vi "Close.vi"(8 "error in (no error)":errorcluster, 11 "DI (N Samples) Ref In":T1) -> (0 "error out":errorcluster)   [LabVIEW 2021, in "DI Block.lvlib"]
doc: "Closes the reference to one or more digital input channels, sets the logic levels of all digital input channels to low, and disables all digital input channels."
uses:
  <vilib>/myRIO/Instrument Drivers/Onboard IO/DI Block/DI Block.lvlib
  <vilib>/myRIO/Instrument Drivers/Onboard IO/DI Block/typedefs/DI Block Reference.ctl
  <vilib>/myRIO/Common/Instrument Driver Framework/Utilities/typedefs/myRIO Generic Hardware Reference.ctl
  <vilib>/myRIO/Common/Instrument Driver Framework/Utilities/typedefs/Hardware Version Enum.ctl
  <vilib>/myRIO/Common/Instrument Driver Framework/Utilities/typedefs/myRIO v1.0 Reference.ctl
  <vilib>/myRIO/Common/Instrument Driver Framework/Utilities/typedefs/Generic FPGA Reference.ctl
  <vilib>/myRIO/Common/Instrument Driver Framework/myRIO v1.0/DI Block/typedefs/DI Block Channels List.ctl
  <vilib>/myRIO/Common/Instrument Driver Framework/myRIO v1.0/DI Block/typedefs/DI Block Channels Enum.ctl
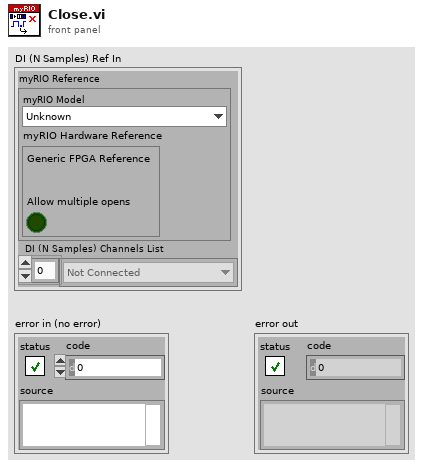
[diagram p1: front panel]
types:
  T1 = typedef "DI Block.lvlib/DI Block Reference.ctl" = cluster{"myRIO Reference":T2, "DI (N Samples) Channels List":T6}
  T2 = typedef "myRIO Generic Hardware Reference.ctl" = cluster{"myRIO Model":T3, "myRIO Hardware Reference":T4}
  T3 = typedef "Hardware Version Enum.ctl" = enum16{"Unknown", "myRIO-1900", "myRIO-1950", "roboRIO", "NI ELVIS RIO CM", "ELVIS III"}
  T4 = typedef "myRIO v1.0 Reference.ctl" = cluster{"Generic FPGA Reference":T5, "Allow multiple opens":bool}
  T5 = typedef "Generic FPGA Reference.ctl" = refnum<k20>
  T6 = typedef "DI Block Channels List.ctl" = T7[]
  T7 = typedef "DI Block Channels Enum.ctl" = enum16{"Not Connected", "A/DI0 (N Samples)", "A/DI1 (N Samples)", "A/DI2 (N Samples)", "A/DI3 (N Samples)", "A/DI4 (N Samples)", "A/DI5 (N Samples)", "A/DI6 (N Samples)", "A/DI7 (N Samples)", "A/DI8 (N Samples)", "A/DI9 (N Samples)", "A/DI10 (N Samples)", "A/DI11 (N Samples)", "A/DI12 (N Samples)", "A/DI13 (N Samples)", "A/DI14 (N Samples)", "A/DI15 (N Samples)", "A/DI16 (N Samples)", "A/DI17 (N Samples)", "A/DI18 (N Samples)", "A/DI19 (N Samples)", "B/DI0 (N Samples)", "B/DI1 (N Samples)", "B/DI2 (N Samples)", "B/DI3 (N Samples)", "B/DI4 (N Samples)", "B/DI5 (N Samples)", "B/DI6 (N Samples)", "B/DI7 (N Samples)", "B/DI8 (N Samples)", "B/DI9 (N Samples)", "B/DI10 (N Samples)", "B/DI11 (N Samples)", "B/DI12 (N Samples)", "B/DI13 (N Samples)", "B/DI14 (N Samples)", "B/DI15 (N Samples)", "B/DI16 (N Samples)", "B/DI17 (N Samples)", "B/DI18 (N Samples)", "B/DI19 (N Samples)"}
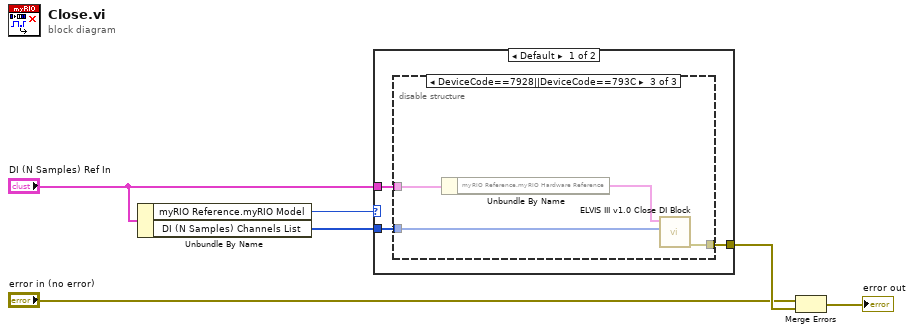
[diagram p0: block diagram]
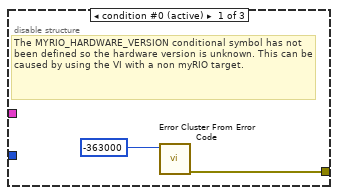
[diagram p2: hidden frame]
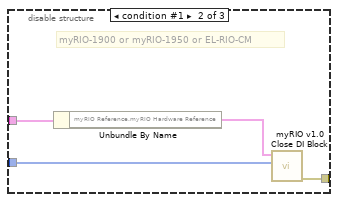
[diagram p3: hidden frame]
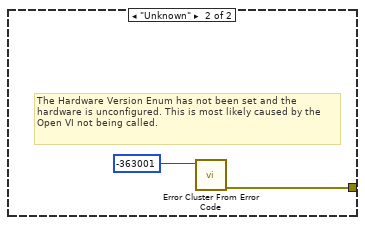
[diagram p4: hidden frame]
diagram:
  n1 = Unbundle By Name("DI (N Samples) Ref In") -> ("myRIO Reference.myRIO Model"=w2:T3, "DI (N Samples) Channels List"=w1:T6)
  n2 = case shown="Default" w2 {
    tunnel: "DI (N Samples) Ref In" -> [w9 _]
    tunnel: [w8 w20] -> w6
    tunnel: w1 -> [w7 _]
    frame Default {
      n3 = disable-structure shown="DeviceCode==7928||DeviceCode==793C" {
        disable-tunnel: w9 -> [_ w15 w18]
        disable-tunnel: [w10 w14 w16] -> w8
        disable-tunnel: w7 -> [_ w12 w17]
        frame condition #0 (active) {
          # "The MYRIO_HARDWARE_VERSION conditional symbol has not been defined so the hardware version is unknown. This can be caused by using the VI with a non myRIO target."
          n4 = call <vilib>:"Error Cluster From Error Code.vi"("error code (0)"=-363000) -> ("error out"=w10:errorcluster)  [unwired: 8 in]
        }
        frame condition #1 {
          # "myRIO-1900 or myRIO-1950 or EL-RIO-CM"
          n5 = Unbundle By Name(w15) -> ("myRIO Reference.myRIO Hardware Reference"=w13:T4)
          n6 = call <vilib>:"myRIO v1.0 Close DI Block.vi"("DI (N Samples) Channel List"=w12, "myRIO Ref In"=w13) -> ("error out"=w14:errorcluster)  [unwired: 9 in]
        }
        frame condition #2 {
          n7 = Unbundle By Name(w18) -> ("myRIO Reference.myRIO Hardware Reference"=w19:T4)
          n8 = call <vilib>:"ELVIS III v1.0 Close DI Block.vi"("DI (N Samples) Channel List"=w17, "myRIO Ref In"=w19) -> ("error out"=w16:errorcluster)  [unwired: 9 in]
        }
      }
    }
    frame "Unknown" {
      # "The Hardware Version Enum has not been set and the hardware is unconfigured. This is most likely caused by the Open VI not being called."
      n9 = call <vilib>:"Error Cluster From Error Code.vi"("error code (0)"=-363001) -> ("error out"=w20:errorcluster)  [unwired: 8 in]
    }
  }
  n10 = Merge Errors("error in (no error)", w6) -> (→"error out":errorcluster)
